vi "GFITS_PostNewFits.vi"(4 "filemsg":string, 6 "before_expID":string="_undef_", 8 "error in":errorcluster, 9 "expID":string="_undef_", 10 "image name":string, 11 "Database RefNum in":T1) -> (2 "message":string)   [LabVIEW 2016]
uses:
  DBSHAND/private/vis/DatabaseHand_RefNum.ctl
  DBSHAND/private/vis/DatabaseHand_Element_Get(string).vi
  DBSHAND/private/vis/DatabaseHand_Element_Set(string).vi
panel:
  in  "cmd struct":T2
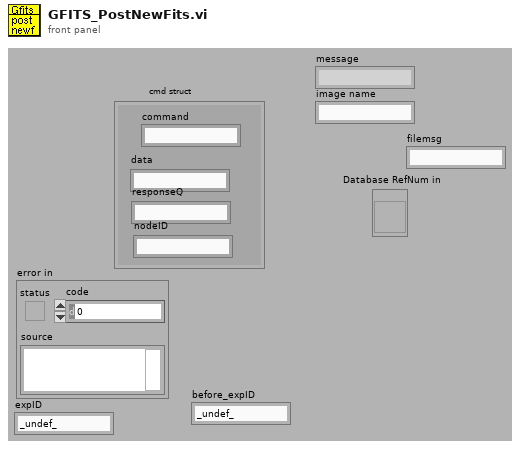
[diagram p1: front panel]
types:
  T1 = typedef "DatabaseHand_RefNum.ctl" = refnum<vi>
  T2 = cluster{"command":string, "data":string, "responseQ":string, "nodeID":string}
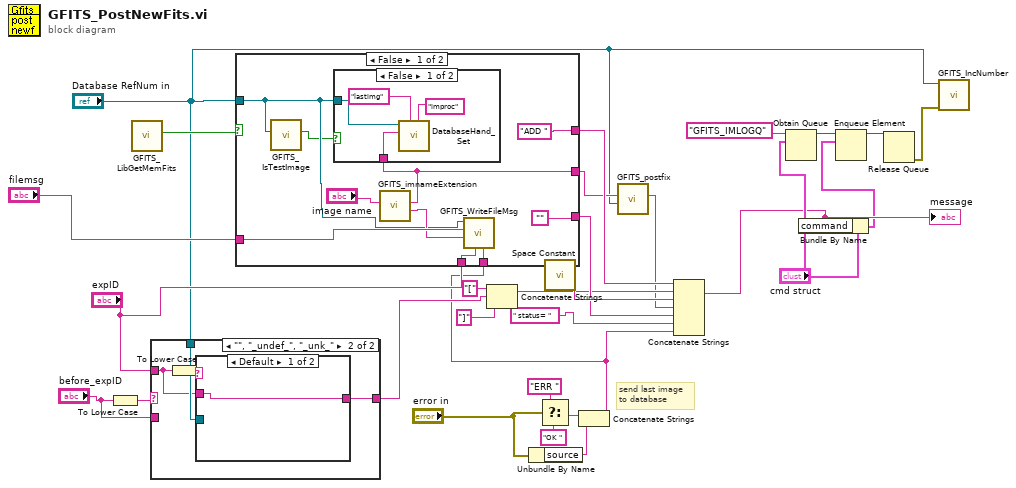
[diagram p0: block diagram]
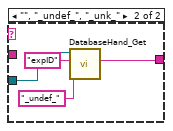
[diagram p3: hidden frame]
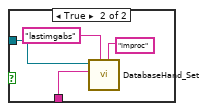
[diagram p4: hidden frame]
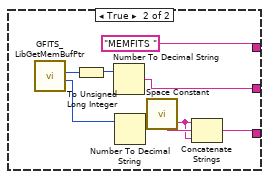
[diagram p5: hidden frame]
diagram:
  # "send last image\nto database"
  n1 = To Lower Case(string="before_expID") -> (all lower case string=w9:string)
  n2 = call "GFITS_LibGetMemFits.vi"() -> ("memfits"=w18:bool)  [unwired: 1 in, 10 out]
  n3 = case shown="\"\", \"_undef_\", \"_unk_\"" w9 {
    tunnel: "expID" -> [_ w31]
    tunnel: [w30 w34] -> w10
    tunnel: "Database RefNum in" -> [_ w33]
    tunnel: "before_expID" -> [w30 _]
    frame Default {
    }
    frame "", "_undef_", "_unk_" {
      n4 = To Lower Case(string=w31) -> (all lower case string=w32:string)
      n5 = case shown="Default" w32 {
        tunnel: [w35 w36] -> w34
        tunnel: w33 -> [_ w39]
        tunnel: w31 -> [w35 _]
        frame Default {
        }
        frame "", "_undef_", "_unk_" {
          n6 = call-poly "DatabaseHand_Get.vi"("default value"="_undef_", "name"="expID", "Database RefNum in"=w39) -> ("value"=w36:string)  [unwired: 2 in, 6 out]
        }
      }
    }
  }
  n7 = Concatenate Strings("[" ("string"), w10, "]" ("string")) -> (w13:string)
  n8 = Unbundle By Name("error in") -> ("source"=w26:string)
  n9 = Select(t="ERR ", s="error in", f="OK ") -> (s? t:f=w27:string)
  n10 = call <vilib>:"Space Constant.vi"() -> ("String"=w16:string)
  n11 = Concatenate Strings(w27, w26) -> (w5:string)
  n12 = case shown="False" w18 {
    tunnel: ["ADD " ("command") "MEMFITS " ("command")] -> w17
    tunnel: [w46 w63] -> w4
    tunnel: "Database RefNum in" -> [w41 _]
    tunnel: ["" w58] -> w15
    tunnel: "filemsg" -> [w45 _]
    tunnel: "expID" -> [w43 _]
    tunnel: w5 -> [w42 _]
    frame False {
      n13 = call "GFITS_IsTestImage.vi"("Database RefNum in"=w41) -> ("testonly"=w40:bool)  [unwired: 10 out]
      n14 = call "GFITS_imnameExtension.vi"("imname in"="image name") -> ("rootname (no extension)"=w44:string, "imname out"=w46:string)  [unwired: 8 out]
      n15 = case shown="False" w40 {
        tunnel: w46 -> [w52 w54]
        tunnel: w41 -> [w50 w55]
        frame False {
          n16 = call-poly "DatabaseHand_Set.vi"("group"="improc", "name"="lastimg", "value"=w52, "Database RefNum in"=w50) -> ()  [unwired: 4 in, 4 out]
        }
        frame True {
          n17 = call-poly "DatabaseHand_Set.vi"("group"="improc", "name"="lastimgabs", "value"=w54, "Database RefNum in"=w55) -> ()  [unwired: 4 in, 4 out]
        }
      }
      n18 = call "GFITS_WriteFileMsg.vi"("status"=w42, "expID"=w43, "image name (no ext)"=w44, "filemsg"=w45, "Database RefNum"=w41) -> ()  [unwired: 1 in, 6 out]
    }
    frame True {
      n19 = call "GFITS_LibGetMemBufPtr.vi"() -> ("fitssize"=w61:i32, "memptr"=w65:u64)  [unwired: 1 in, 9 out]
      n20 = To Unsigned Long Integer(number=w65) -> (unsigned 32bit integer=w64:u32)
      n21 = Number To Decimal String(number=w64) -> (decimal integer string=w63:string)  [unwired: 1 out]
      n22 = Number To Decimal String(number=w61) -> (decimal integer string=w60:string)  [unwired: 1 out]
      n23 = call <vilib>:"Space Constant.vi"() -> ("String"=w59:string)
      n24 = Concatenate Strings(w59, w60, w59) -> (w58:string)
    }
  }
  n25 = call "GFITS_postfix.vi"("Database RefNum in"="Database RefNum in", "imname in"=w4) -> ("imname out"=w3:string)  [unwired: 9 out]
  n26 = Concatenate Strings(w17, w13, w16, w3, w15, " status= " ("string"), w5) -> (w21:string)
  "message" <- w21
  n27 = Obtain Queue(name (unnamed)="GFITS_IMLOGQ", element data type="cmd struct") -> (queue out=w24:refnum<queue>)  [unwired: 3 in, 2 out]
  n28 = Bundle By Name(cluster="cmd struct", "command"=w21) -> (w20:T2)
  n29 = Enqueue Element(queue=w24, element=w20) -> (queue out=w23:refnum<queue>)  [unwired: 1 in, 3 out]
  n30 = Release Queue(queue=w23) -> (error out=w2:errorcluster)  [unwired: 1 in, 3 out]
  n31 = call "GFITS_IncNumber.vi"("error in (no error)"=w2, "Database RefNum"="Database RefNum in") -> ()  [unwired: 10 out]
